vi "Generate SQL Values.vi"(8 "error in (no error)":errorcluster, 11 "Banking Record in":refnum<class "Banking Transaction.lvclass">) -> (0 "error out":errorcluster, 2 "SQL Values":string, 3 "Banking Record out":refnum<class "Banking Transaction.lvclass">)   [LabVIEW 2018, in "Banking Transaction.lvclass"]
uses:
  Banking Transaction.lvclass
  Banking Transaction.lvclass/Banking Transaction.ctl
  Transaction/Transaction.lvclass
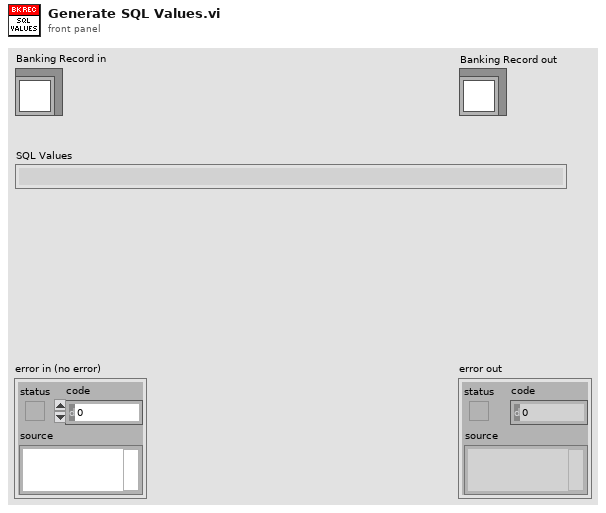
[diagram p1: front panel]
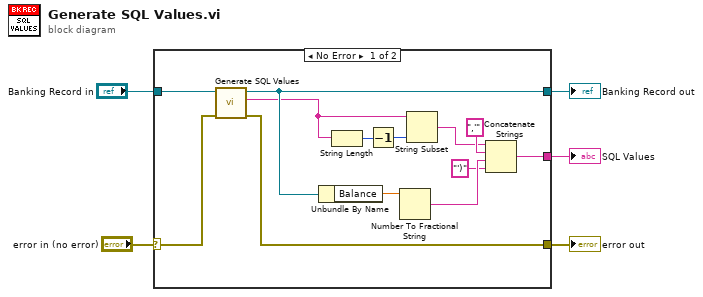
[diagram p0: block diagram]
diagram:
  n1 = case shown="No Error" "error in (no error)" {
    selector: "error in (no error)" -> [w16 w20]
    tunnel: [w18 w20] -> w5
    tunnel: [w11 _] -> w4
    tunnel: [w15 w19] -> w3
    tunnel: "Banking Record in" -> [w17 w19]
    frame No Error {
      n2 = call-parent "Generate SQL Values.vi"("error in (no error)"=w16, "Transaction in"=w17) -> ("error out"=w18:errorcluster, "SQL Values"=w8:string, "Transaction out"=w15:refnum<class "Banking Transaction.lvclass">)  [unwired: 7 in]
      n3 = Unbundle By Name(w15) -> ("Balance"=w14:dbl)
      n4 = String Length(string=w8) -> (length=w9:i32)
      n5 = Decrement(x=w9) -> (x-1=w7:i32)
      n6 = Number To Fractional String(number=w14) -> (F-format string=w12:string)  [unwired: 3 in]
      n7 = String Subset(string=w8, length (rest)=w7) -> (substring=w6:string)  [unwired: 1 in]
      n8 = Concatenate Strings(w6, ",'" ("string"), w12, "')" ("string")) -> (w11:string)
    }
    frame Error {
    }
  }
  "error out" <- w5
  "Banking Record out" <- w3
  "SQL Values" <- w4
